vi "Get Software Version.vi"(11 "Data":string) -> (0 "Daily Revision":string, 1 "Non-Critical Major":string, 2 "Critical Minor":string, 3 "Critical Major":string, 4 "Non-Critical Minor":string)   [LabVIEW 2016, in "GEA2_Toolkit.lvlib"]
uses:
  library/GEA2_Toolkit.lvlib
panel:
  # "01 0A 03 05"
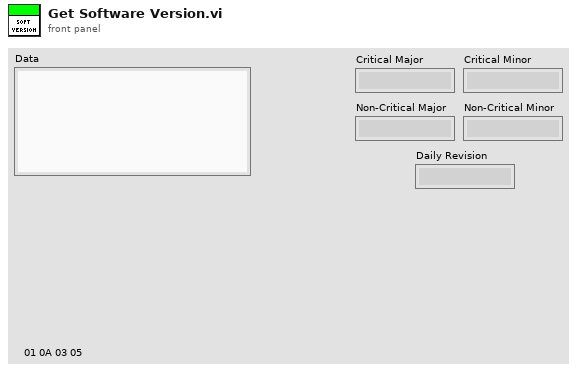
[diagram p1: front panel]
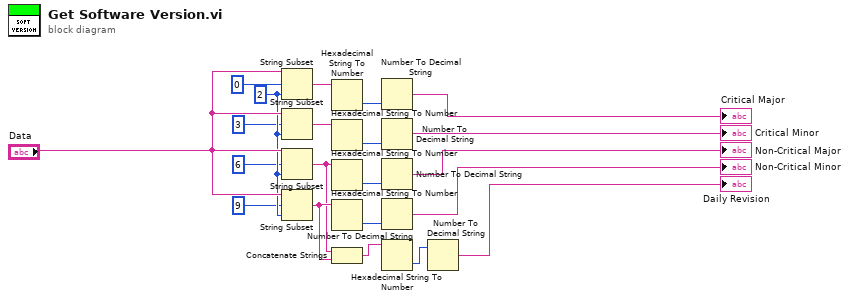
[diagram p0: block diagram]
diagram:
  w15 = 2 ("length (rest)")
  n1 = String Subset(string="Data", offset (0)=0 ("length (rest)"), length (rest)=w15) -> (substring=w1:string)
  n2 = String Subset(string="Data", offset (0)=3 ("length (rest)"), length (rest)=w15) -> (substring=w5:string)
  n3 = String Subset(string="Data", offset (0)=6 ("length (rest)"), length (rest)=w15) -> (substring=w10:string)
  n4 = String Subset(string="Data", offset (0)=9 ("length (rest)"), length (rest)=w15) -> (substring=w11:string)
  n5 = Hexadecimal String To Number(string=w1) -> (number=w6:u32)  [unwired: 2 in, 1 out]
  n6 = Hexadecimal String To Number(string=w5) -> (number=w7:u32)  [unwired: 2 in, 1 out]
  n7 = Hexadecimal String To Number(string=w10) -> (number=w8:u32)  [unwired: 2 in, 1 out]
  n8 = Hexadecimal String To Number(string=w11) -> (number=w9:u32)  [unwired: 2 in, 1 out]
  n9 = Concatenate Strings(w10, w11) -> (w12:string)
  n10 = Number To Decimal String(number=w6) -> (decimal integer string=→"Critical Major":string)  [unwired: 1 in]
  n11 = Number To Decimal String(number=w7) -> (decimal integer string=→"Critical Minor":string)  [unwired: 1 in]
  n12 = Number To Decimal String(number=w8) -> (decimal integer string=→"Non-Critical Major":string)  [unwired: 1 in]
  n13 = Number To Decimal String(number=w9) -> (decimal integer string=→"Non-Critical Minor":string)  [unwired: 1 in]
  n14 = Hexadecimal String To Number(string=w12) -> (number=w13:u32)  [unwired: 2 in, 1 out]
  n15 = Number To Decimal String(number=w13) -> (decimal integer string=→"Daily Revision":string)  [unwired: 1 in]
